vi "Array Add or Remove.vi"(10 "Size":i32, 11 "Array in":dbl[](array[numeric])) -> (3 "Arry out":dbl[](array[numeric]))   [LabVIEW 2016, in "Instrument.Lockin.lvclass"]
uses:
  Instrument.Lockin.lvclass
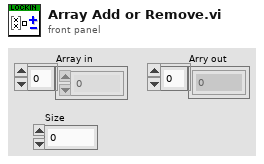
[diagram p1: front panel]
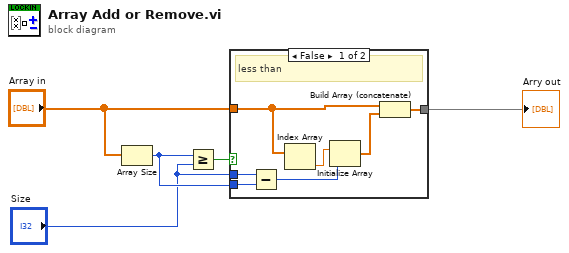
[diagram p0: block diagram]
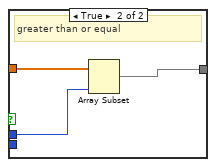
[diagram p2: hidden frame]
diagram:
  n1 = Array Size(array="Array in") -> (size(s)=w5:i32)
  n2 = Greater Or Equal?(x=w5, y="Size") -> (x >= y?=w3:bool)
  n3 = case shown="False" w3 {
    tunnel: "Array in" -> [w6 w15]
    tunnel: "Size" -> [w9 w14]
    tunnel: [w10 w13] -> w2
    tunnel: w5 -> [w8 _]
    frame False {
      # "less than"
      n4 = Subtract(x=w9, y=w8) -> (x-y=w7:i32)
      n5 = Index Array(array=w6) -> (element=w11:dbl)  [unwired: 1 in]
      n6 = Initialize Array(w11, w7) -> (w12:dbl[])
      n7 = Build Array (concatenate)(w6, w12) -> (w10:dbl[])
    }
    frame True {
      # "greater than or equal"
      n8 = Array Subset(array=w15, length=w14) -> (w13:dbl[])  [unwired: 1 in]
    }
  }
  "Arry out" <- w2
